vi "CheckFlame Choose State.vi"(7 "State String":string, 8 "error in":errorcluster, 10 "Timer Outputs":T1, 11 "Queue in":refnum<queue>) -> (0 "error out":errorcluster, 2 "String":string, 3 "Queue out":refnum<queue>)   [LabVIEW 2013]
doc: "This sub-VI determines which states to call next based on the status of the SVM timer FGV."
uses:
  Controls/timer_output_cluster.ctl
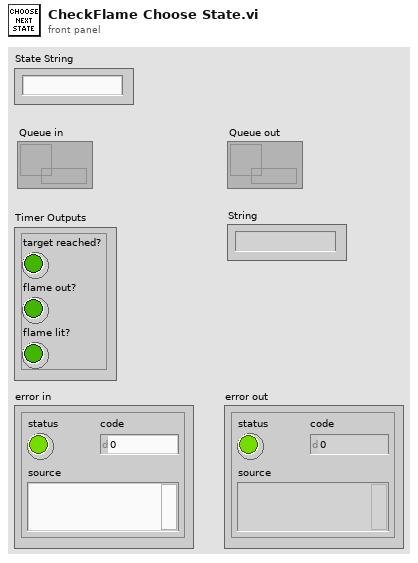
[diagram p1: front panel]
types:
  T1 = typedef "timer_output_cluster.ctl" = cluster{"target reached?":bool, "flame out?":bool, "flame lit?":bool}
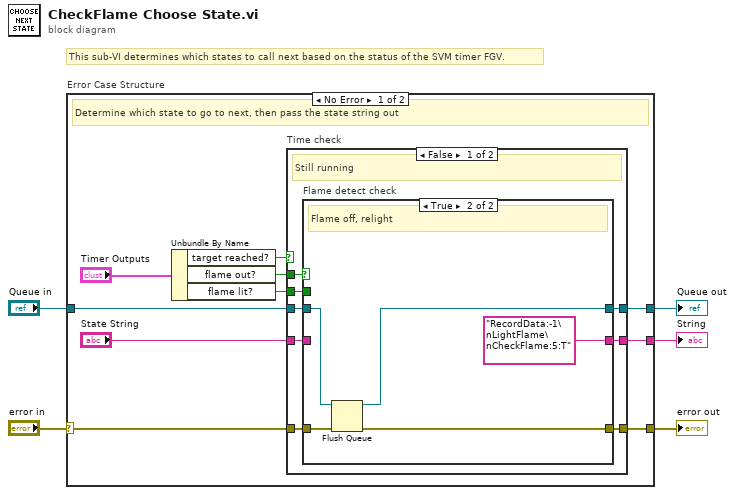
[diagram p0: block diagram]
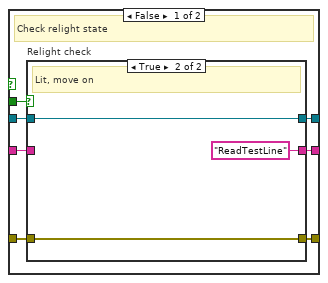
[diagram p2: hidden frame]
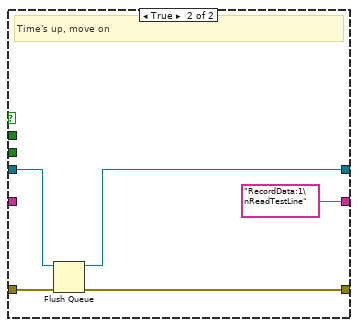
[diagram p4: hidden frame]
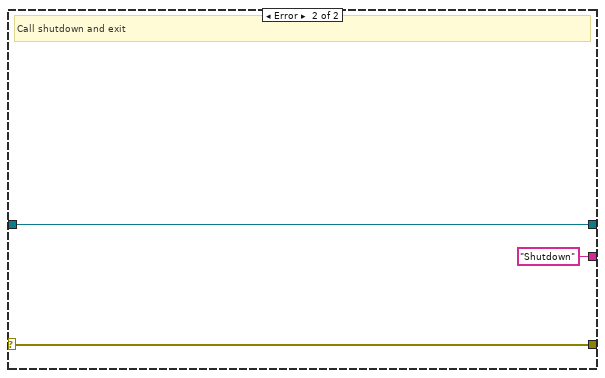
[diagram p5: hidden frame]
diagram:
  # "This sub-VI determines which states to call next based on the status of the SVM timer FGV."
  n1 = case "Error Case Structure" shown="No Error" "error in" {
    selector: "error in" -> [w9 w49]
    tunnel: "Queue in" -> [w12 w47]
    tunnel: [w11 "Shutdown"] -> w4
    tunnel: [w10 w49] -> w3
    tunnel: [w8 w47] -> w1
    frame No Error {
      # "Determine which state to go to next, then pass the state string out"
      n2 = Unbundle By Name("Timer Outputs") -> ("target reached?"=w13:bool, "flame out?"=w14:bool, "flame lit?"=w15:bool)
      n3 = case "Time check" shown="False" w13 {
        tunnel: [w23 w45] -> w10
        tunnel: [w22 "RecordData:1\nReadTestLine"] -> w11
        tunnel: w12 -> [w21 w44]
        tunnel: [w20 w43] -> w8
        tunnel: w14 -> [w19 _]
        tunnel: w15 -> [w18 _]
        tunnel: w9 -> [w17 w42]
        tunnel: "State String" -> [w16 _]
        frame False {
          # "Still running"
          n4 = case "Flame detect check" shown="True" w19 {
            tunnel: [w25 w40] -> w23
            tunnel: [w30 "RecordData:-1\nLightFlame\nCheckFlame:5:T"] -> w22
            tunnel: w21 -> [w29 w39]
            tunnel: [w27 w38] -> w20
            tunnel: w18 -> [w28 _]
            tunnel: w17 -> [w26 w37]
            tunnel: w16 -> [w24 _]
            frame False {
              # "Check relight state"
              n5 = case "Relight check" shown="True" w28 {
                tunnel: [w31 "ReadTestLine"] -> w30
                tunnel: w29 -> [w33 w36]
                tunnel: [w33 w36] -> w27
                tunnel: w26 -> [w32 w34]
                tunnel: [w32 w34] -> w25
                tunnel: w24 -> [w31 _]
                frame False {
                  # "Repeat current state"
                }
                frame True {
                  # "Lit, move on"
                }
              }
            }
            frame True {
              # "Flame off, relight"
              n6 = Flush Queue(queue=w39, error in (no error)=w37) -> (queue out=w38:refnum<queue>, error out=w40:errorcluster)  [unwired: 1 out]
            }
          }
        }
        frame True {
          # "Time's up, move on"
          n7 = Flush Queue(queue=w44, error in (no error)=w42) -> (queue out=w43:refnum<queue>, error out=w45:errorcluster)  [unwired: 1 out]
        }
      }
    }
    frame Error {
      # "Call shutdown and exit"
    }
  }
  "String" <- w4
  "error out" <- w3
  "Queue out" <- w1
